vi "Update Metric.vi"(6 "Period s (1)":dbl=1.0, 7 "Metric":string, 8 "error in (no error)":errorcluster, 10 "Value":dbl, 11 "Module in":refnum<class "Module.lvclass">) -> (0 "error out":errorcluster, 3 "Module out":refnum<class "Module.lvclass">)   [LabVIEW 2020, in "Volatus.lvlib" / "Module.lvclass"]
uses:
  Module.lvclass
  Metric Update.ctl
  Module.lvclass/Module.ctl
  MessageQ/MessageQ.lvclass/MessageQ.ctl
  Parent Q.vi
  MessageQ/Is Null.vi
  MessageQ/Send.vi
  Volatus.lvlib
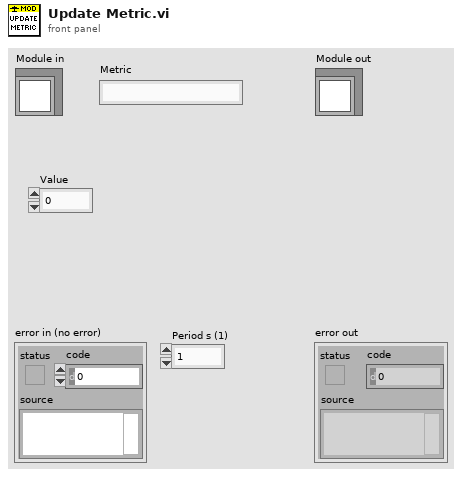
[diagram p1: front panel]
types:
  T1 = typedef "Volatus.lvlib/Metric Update.ctl" = cluster{"Hierarchy":string[], "Name":string, "Value":dbl}
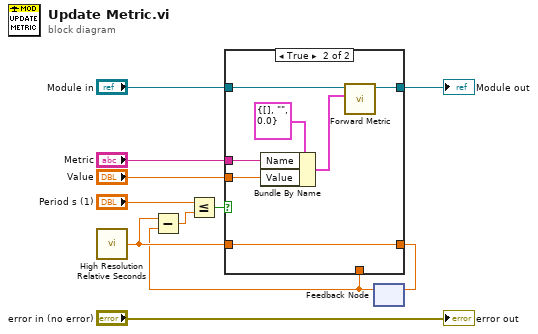
[diagram p0: block diagram]
diagram:
  n1 = call <vilib>:"High Resolution Relative Seconds.vi"() -> ("relative seconds"=w4:dbl)
  n2 = feedback #1() -> (w2:dbl)  [unwired: 1 in]
  n3 = Subtract(x=w4, y=w2) -> (x-y=w3:dbl)
  n4 = Less Or Equal?(x="Period s (1)", y=w3) -> (x <= y?=w5:bool)
  n5 = case shown="True" w5 {
    tunnel: "Module in" -> [w12 w20]
    tunnel: "Metric" -> [_ w18]
    tunnel: "Value" -> [_ w17]
    tunnel: [w12 w16] -> w7
    tunnel: w4 -> [_ w14]
    tunnel: w2 -> [w13 _]
    tunnel: [w13 w14] -> w1
    frame False {
    }
    frame True {
      n6 = Bundle By Name(cluster=T1 {"Hierarchy"=[], "Name"="", "Value"=0.0} ("Metric Update"), "Name"=w18, "Value"=w17) -> (w15:T1)
      n7 = call "Forward Metric.vi"("Metric Update"=w15, "Module in"=w20) -> ("Module out"=w16:refnum<class "Module.lvclass">)  [unwired: 8 in, 1 out]
    }
  }
  "Module out" <- w7
  n8 = feedback-in #1(w1) -> ()
  "error out" <- "error in (no error)"
